vi "Get Name.vi"(11 "Game in":refnum<class "Game.lvclass">) -> (2 "Name":string)   [LabVIEW 2020, in "Conditum-Example.lvlib" / "Game.lvclass"]
uses:
  Game.lvclass
  Conditum/Columns/String/String.lvclass
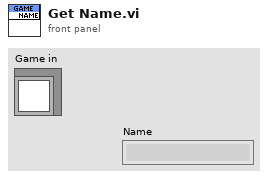
[diagram p1: front panel]
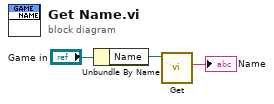
[diagram p0: block diagram]
diagram:
  n1 = Unbundle By Name("Game in") -> ("Name"=w2:refnum<class "String.lvclass">)
  n2 = call "Get.vi"("String in"=w2) -> ("Value"=→"Name":string)  [unwired: 10 in]
